vi "Read Value.vi"(8 "error in (no error)":errorcluster, 9 "timeout in ms (-1)":i32=-1, 11 "Future in":refnum<class "Future.lvclass">) -> (0 "error out":errorcluster, 1 "timed out?":bool, 2 "Value":variant)   [LabVIEW 2017, in "Promise Future.lvlib" / "Future.lvclass"]
uses:
  Future.lvclass
  Future.lvclass/Future.ctl
  Rejected Future/Rejected Future.lvclass/Rejected Future.ctl
  <vilib>/Utility/error.llb/Error Cluster From Error Code.vi
  <vilib>/ErrorRing/Error Ring.xnode
  Rejected Future/Rejected Future.lvclass
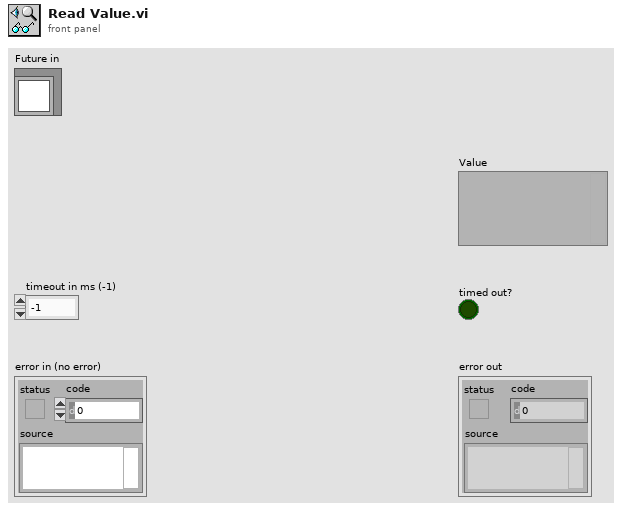
[diagram p1: front panel]
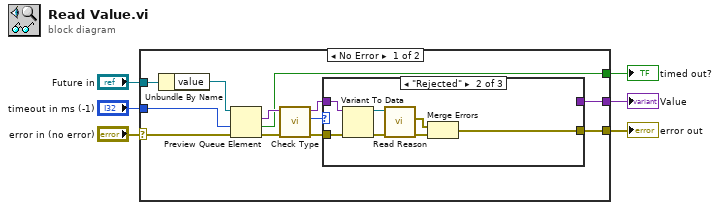
[diagram p0: block diagram]
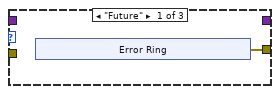
[diagram p2: hidden frame]
diagram:
  n1 = case shown="No Error" "error in (no error)" {
    selector: "error in (no error)" -> [w14 w34]
    tunnel: [w17 w34] -> w2
    tunnel: "Future in" -> [w15 _]
    tunnel: [w7 _] -> w3
    tunnel: [w18 _] -> w4
    tunnel: "timeout in ms (-1)" -> [w16 _]
    frame No Error {
      n2 = Unbundle By Name(w15) -> ("value"=w11:refnum<queue>)
      n3 = Preview Queue Element(queue=w11, timeout in ms (-1)=w16, error in (no error)=w14) -> (element=w13:variant, timed out?=w7:bool, error out=w12:errorcluster)  [unwired: 1 out]
      n4 = call "Check Type.vi"("error in"=w12, "Value in"=w13) -> ("error out"=w10:errorcluster, "Type"=w9:enum16{"Value", "Future", "Rejected"}, "Value out"=w8:variant)  [unwired: 7 in]
      n5 = case shown="\"Rejected\"" w9 {
        tunnel: [_ _ w32] -> w18
        tunnel: w10 -> [_ w31 w33]
        tunnel: [w19 w26 w33] -> w17
        tunnel: w8 -> [_ w28 w32]
        frame "Future" {
          # "Future was resolved with another future"
          n6 = xnode "Error Ring"() -> ("error out"=w19:errorcluster)
        }
        frame "Rejected" {
          n7 = Variant To Data(error in=w31, Variant=w28) -> (data=w29:refnum<class "Rejected Future.lvclass">, error out=w30:errorcluster)  [unwired: 1 in]
          n8 = call "Read Reason.vi"("error in (no error)"=w30, "Rejected Future in"=w29) -> ("error out"=w27:errorcluster, "Reason"=w25:errorcluster)  [unwired: 7 in, 1 out]
          n9 = Merge Errors(w25, w27) -> (w26:errorcluster)
        }
        frame "Value" {
          # "Just a normal value, pass it along"
        }
      }
    }
    frame Error {
    }
  }
  "error out" <- w2
  "Value" <- w4
  "timed out?" <- w3
